vi "Add Entry.vi"(7 "severity":i32(ring)=2 caption="severity (Error)" items=["Error", "Warning", "Informational"], 8 "error in (no error)":errorcluster, 9 "Data":variant, 10 "Origin":string, 11 "Logging in":refnum<class "Logging.lvclass">) -> (0 "error out":errorcluster, 3 "Logging out":refnum<class "Logging.lvclass">)   [LabVIEW 2020, in "Logging.lvclass"]
uses:
  Logging.lvclass
  Logging.lvclass/Logging.ctl
  controls/Log entry.ctl
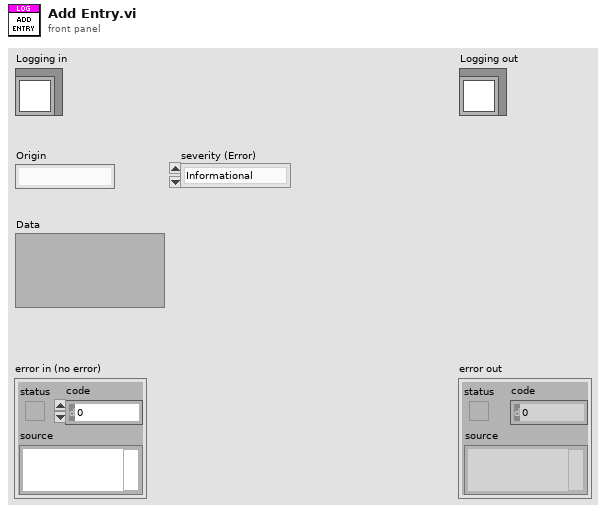
[diagram p1: front panel]
types:
  T1 = typedef "Log entry.ctl" = cluster{"timestamp":timestamp, "data":variant, "origin":string, "severity":i32}
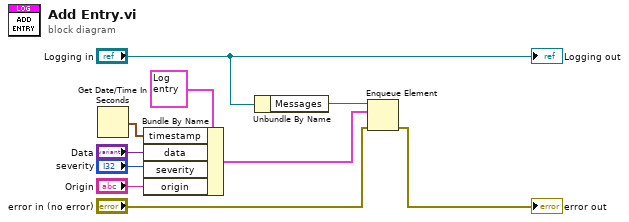
[diagram p0: block diagram]
diagram:
  n1 = Get Date/Time In Seconds() -> (seconds since 1Jan1904=w2:timestamp)
  n2 = Bundle By Name(cluster=T1 {"timestamp"=timestamp(0 s since 1904-01-01), "data"=variant, "origin"="", "severity"=0} ("Log entry"), "timestamp"=w2, "data"="Data", "severity"="severity", "origin"="Origin") -> (w1:T1)
  n3 = Unbundle By Name("Logging in") -> ("Messages"=w4:refnum<queue>)
  n4 = Enqueue Element(queue=w4, element=w1, error in (no error)="error in (no error)") -> (error out=→"error out":errorcluster)  [unwired: 1 in, 2 out]
  "Logging out" <- "Logging in"
